vi "Initialise.vi"   [LabVIEW 2019]
uses:
  <vilib>/myRIO/Instrument Drivers/Onboard IO/DIO/typedefs/DIO Reference.ctl
  <vilib>/myRIO/Common/Instrument Driver Framework/Utilities/typedefs/myRIO Generic Hardware Reference.ctl
  <vilib>/myRIO/Common/Instrument Driver Framework/Utilities/typedefs/Hardware Version Enum.ctl
  <vilib>/myRIO/Common/Instrument Driver Framework/Utilities/typedefs/myRIO v1.0 Reference.ctl
  <vilib>/myRIO/Common/Instrument Driver Framework/Utilities/typedefs/Generic FPGA Reference.ctl
  <vilib>/myRIO/Common/Instrument Driver Framework/myRIO v1.0/DIO/typedefs/DIO Channels List.ctl
  <vilib>/myRIO/Common/Instrument Driver Framework/myRIO v1.0/DIO/typedefs/DIO Channels Enum.ctl
  <vilib>/userDefined/High Color/nirio_resource_hc.ctl
  <vilib>/myRIO/Common/Instrument Driver Framework/Utilities/vis/Is FPGA Ref Available.vi
  <vilib>/myRIO/Common/Instrument Driver Framework/myRIO v1.0/DIO/vis/myRIO v1.1 Open DIO.vi
  <vilib>/myRIO/Instrument Drivers/Onboard IO/DIO/vis/Write.vi
  <vilib>/myRIO/Common/Instrument Driver Framework/Utilities/vis/Validate Channels.vi
  <vilib>/myRIO/Common/Instrument Driver Framework/myRIO v1.0/DIO/vis/myRIO v1.0 Reserve DIO.vi
  <vilib>/myRIO/Common/Instrument Driver Framework/myRIO v1.0/Resource Manager/vis/myRIO v1.0 Reserve Channel List.vi
  <vilib>/myRIO/Common/Instrument Driver Framework/myRIO v1.0/DIO/vis/myRIO v1.0 Build MUX Configuration DIO.vi
  <vilib>/myRIO/Common/Instrument Driver Framework/myRIO v1.0/Resource Manager/vis/myRIO v1.0 Reserve Channel.vi
  <vilib>/myRIO/Common/Instrument Driver Framework/myRIO v1.0/Resource Manager/vis/myRIO v1.0 Unreserve Channel.vi
  <vilib>/myRIO/Common/Instrument Driver Framework/myRIO v1.0/Resource Manager/vis/myRIO v1.0 Create Configuration List.vi
  <vilib>/myRIO/Common/Instrument Driver Framework/myRIO v1.0/Resource Manager/vis/myRIO v1.0 Build Mutex Name.vi
  <vilib>/Utility/VariantDataType/GetNumericInfo.vi
  <vilib>/Utility/error.llb/Error Cluster From Error Code.vi
  <vilib>/myRIO/Common/Instrument Driver Framework/myRIO v1.0/myRIO v1.1 Open.vi
  <vilib>/myRIO/Common/Instrument Driver Framework/Utilities/vis/IO Manager.vi
  <vilib>/myRIO/Common/Instrument Driver Framework/Utilities/vis/Configuration Manager.vi
  <vilib>/myRIO/Common/Instrument Driver Framework/myRIO v1.0/Resource Manager/vis/myRIO v1.0 Configure IO.vi
  <vilib>/myRIO/Common/Instrument Driver Framework/myRIO v1.0/myRIO v1.0 Close.vi
  <vilib>/myRIO/Common/Instrument Driver Framework/myRIO v1.0/DIO/vis/myRIO v1.0 Write DIO.vi
  <vilib>/myRIO/Express VI/Onboard Devices/LED/LED Express VI.xnode
  <vilib>/myRIO/Instrument Drivers/Onboard IO/DIO/vis/myRIO DIO Open.xnode
  <vilib>/myRIO/Express VI/Onboard IO/DO/DO Express VI.xnode
  <vilib>/myRIO/Instrument Drivers/Onboard IO/DIO/DIO.lvlib
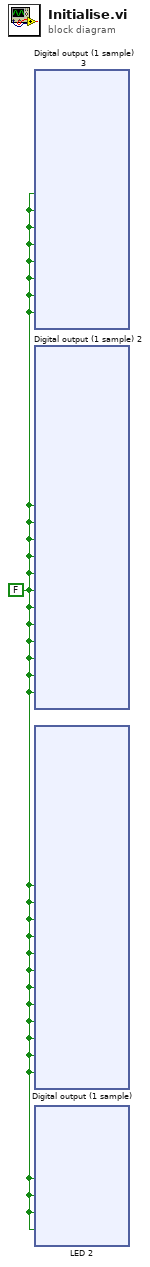
[diagram p0: block diagram]
diagram:
  w1 = FALSE
  n1 = xnode "Digital output (1 sample) 3"("B/DIO8 (Pin 27)"=w1, "B/DIO9 (Pin 29)"=w1, "B/DIO10 (Pin 31)"=w1, "B/DIO11 (Pin 18)"=w1, "B/DIO12 (Pin 22)"=w1, "B/DIO13 (Pin 26)"=w1, "B/DIO14 (Pin 32)"=w1, "B/DIO15 (Pin 34)"=w1) -> ()  [unwired: 1 in, 1 out]
  n2 = xnode "Digital output (1 sample) 2"("A/DIO12 (Pin 22)"=w1, "A/DIO13 (Pin 26)"=w1, "A/DIO14 (Pin 32)"=w1, "A/DIO15 (Pin 34)"=w1, "B/DIO0 (Pin 11)"=w1, "B/DIO1 (Pin 13)"=w1, "B/DIO2 (Pin 15)"=w1, "B/DIO3 (Pin 17)"=w1, "B/DIO4 (Pin 19)"=w1, "B/DIO5 (Pin 21)"=w1, "B/DIO6 (Pin 23)"=w1, "B/DIO7 (Pin 25)"=w1) -> ()  [unwired: 1 in, 1 out]
  n3 = xnode "Digital output (1 sample)"("A/DIO0 (Pin 11)"=w1, "A/DIO1 (Pin 13)"=w1, "A/DIO2 (Pin 15)"=w1, "A/DIO3 (Pin 17)"=w1, "A/DIO4 (Pin 19)"=w1, "A/DIO5 (Pin 21)"=w1, "A/DIO6 (Pin 23)"=w1, "A/DIO7 (Pin 25)"=w1, "A/DIO8 (Pin 27)"=w1, "A/DIO9 (Pin 29)"=w1, "A/DIO10 (Pin 31)"=w1, "A/DIO11 (Pin 18)"=w1) -> ()  [unwired: 1 in, 1 out]
  n4 = xnode "LED 2"("LED0"=w1, "LED1"=w1, "LED2"=w1, "LED3"=w1) -> ()  [unwired: 1 in, 1 out]
